vi "DownloadRunMain.vi"(11 "uPythonX":T1={"VISA Refnum in"="", "Python Code"="# Type Code Here"}) -> (0 "error out":errorcluster, 1 "Reply":string, 3 "VISA Refnum out":refnum<visa-resource-name>)   [LabVIEW 2016]
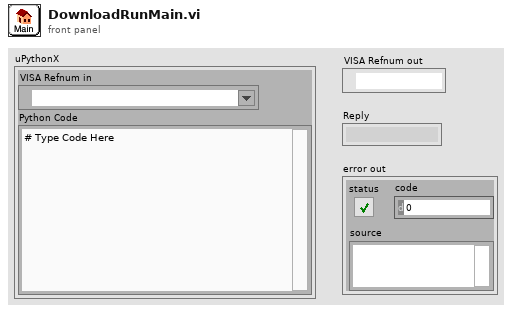
[diagram p1: front panel]
types:
  T1 = cluster{"VISA Refnum in":refnum<visa-resource-name>, "Python Code":string}
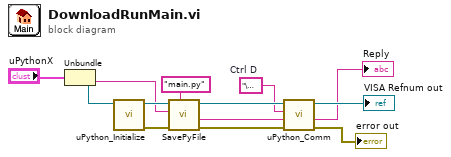
[diagram p0: block diagram]
diagram:
  w7 = "\u0004"  # Ctrl D
  n1 = Unbundle("uPythonX") -> ("VISA Refnum in"=w5:refnum<visa-resource-name>, "Python Code"=w4:string)
  n2 = call "uPython_Initialize.vi"("VISA Refnum in"=w5) -> ("error out"=w12:errorcluster, "VISA Refnum out"=w13:refnum<visa-resource-name>)  [unwired: 9 in]
  n3 = call "SavePyFile.vi"("Name"="main.py", "error in"=w12, "Python Code"=w4, "VISA in"=w13) -> ("error out"=w9:errorcluster, "Reply"=w3:string, "VISA out"=w11:refnum<visa-resource-name>)  [unwired: 5 in]
  n4 = call "uPython_Comm.vi"("error in (no error)"=w9, "Console In"=w3, "Script"=w7, "VISA Refnum in"=w11) -> ("error out"=→"error out":errorcluster, "Console Out"=→"Reply":string, "VISA out"=→"VISA Refnum out":refnum<visa-resource-name>)  [unwired: 3 in, 2 out]
